vi "MeasurementServer_FourProbeMeasurement_WriteValue.vi"(0 "gRPCid":T3, 1 "FourProbeRawData":T1, 3 "error in (no error)":errorcluster) -> (10 "error out":errorcluster)   [LabVIEW 2019, in "labview-grpc-measurement-server.lvlib"]
uses:
  labview-grpc-measurement-server.lvlib
  MeasurementServer_gRPCid.ctl
  MeasurementServer_FourProbeRawData.ctl
  MeasurementServer_ErrorOutData.ctl
  <vilib>/Utility/error.llb/Error Cluster From Error Code.vi
  <vilib>/ErrorRing/Error Ring.xnode
  home/lvuser/liblabview_measurement_server.so
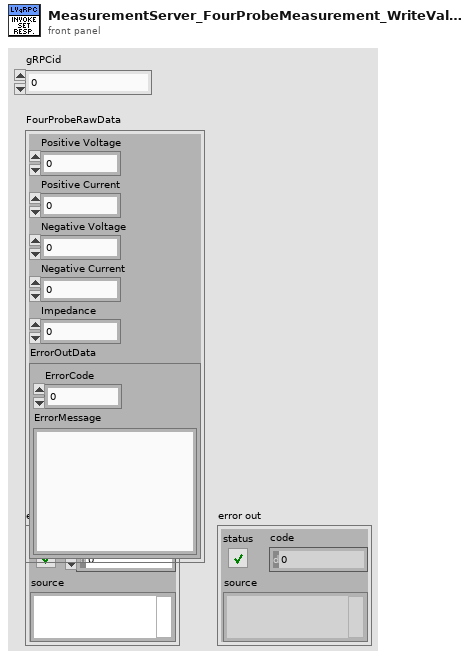
[diagram p1: front panel]
types:
  T1 = typedef "labview-grpc-measurement-server.lvlib/MeasurementServer_FourProbeRawData.ctl" = cluster{"Positive Voltage":dbl, "Positive Current":dbl, "Negative Voltage":dbl, "Negative Current":dbl, "Impedance":dbl, "ErrorOutData":T2}
  T2 = typedef "labview-grpc-measurement-server.lvlib/MeasurementServer_ErrorOutData.ctl" = cluster{"ErrorCode":i32, "ErrorMessage":string}
  T3 = typedef "labview-grpc-measurement-server.lvlib/MeasurementServer_gRPCid.ctl" = u64
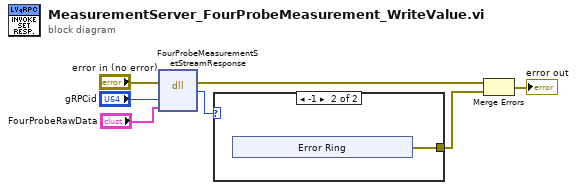
[diagram p0: block diagram]
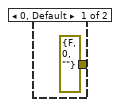
[diagram p2: hidden frame]
diagram:
  n1 = dll-call lib="home/lvuser/liblabview_measurement_server.so" fn="FourProbeMeasurementSetStreamResponse"(error in="error in (no error)", "id"="gRPCid", "data"="FourProbeRawData") -> (error out=w2:errorcluster, "return type"=w4:i32)  [unwired: 4 in, 1 out]
  n2 = case shown="-1" w4 {
    tunnel: [errorcluster {"status"=FALSE, "code"=0, "source"=""} ("error constant") w9] -> w3
    frame 0, Default {
    }
    frame -1 {
      n3 = xnode "Error Ring"() -> ("error out"=w9:errorcluster)
    }
  }
  n4 = Merge Errors(w2, w3) -> (→"error out":errorcluster)
